vi "Parse XML Tree Example.vi"() -> ()   [LabVIEW 2016]
uses:
  <vilib>/xml/Load XML File.vi
  <vilib>/ni/Tree/Tree Manager/API/List Roots.vi
  <vilib>/ni/Tree/Tree Manager/Tree.lvclass
  <vilib>/xml/NI_XML.lvlib
panel:
  in  "Tree":string(tree)
  out "Error Out":errorcluster
  in  "path to XML document":path
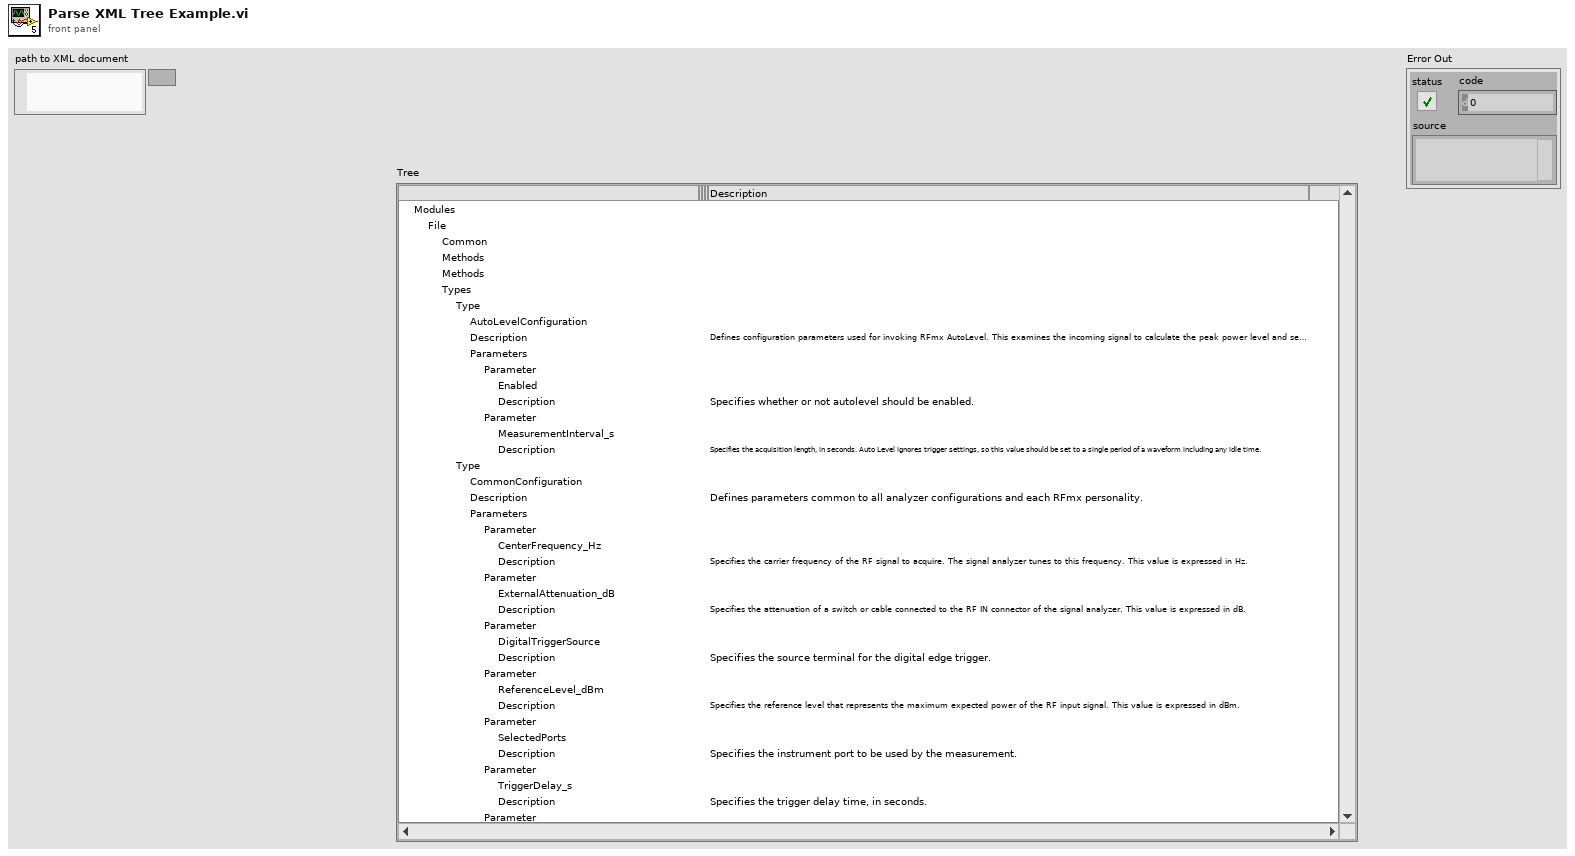
[diagram p1: front panel]
types:
  T1 = cluster{"Left Cell String":string, "Child Text":string[], "Child Tag":string, "Item Indent":i32, "Child Only?":bool, "Glyph Index":i32}[]
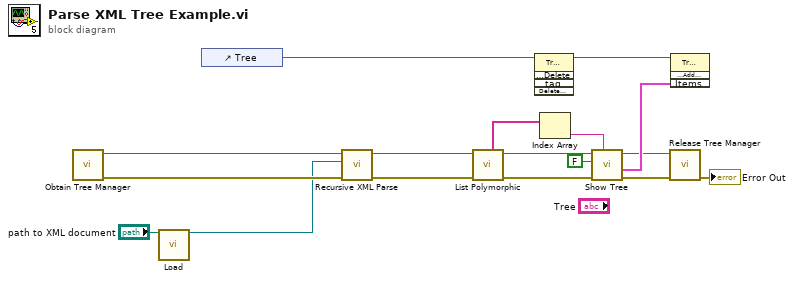
[diagram p0: block diagram]
diagram:
  n1 = call <vilib>:"Obtain Tree Manager.vi"() -> ("Error Out"=w15:errorcluster, "Tree"=w8:refnum<data-value>)  [unwired: 10 in]
  n2 = call-poly <vilib>:"Load.vi"("path to XML document"="path to XML document") -> ("DOM document out"=w1:refnum<k20>)  [unwired: 12 in, 2 out]
  n3 = control-ref of="Tree"() -> (w3:refnum<vi>)
  n4 = call "Recursive XML Parse.vi"("error in (no error)"=w15, "DOM document in"=w1, "Tree"=w8) -> ("error out"=w14:errorcluster, "Tree Manager"=w7:refnum<data-value>)  [unwired: 7 in]
  n5 = call-poly <vilib>:"List Polymorphic.vi"("Error In"=w14, "Tree"=w7) -> ("Error Out"=w13:errorcluster, "Tree"=w12:refnum<data-value>, "Roots IDs"=w4:string[])  [unwired: 6 in, 1 out]
  n6 = invoke class="Tree (strict)" method="Edit Tree Items.Delete"(reference=w3) -> (reference out=w16:refnum<vi>)  [unwired: 4 in, 4 out]
  n7 = Index Array(array=w4) -> (element=w11:string)  [unwired: 1 in]
  n8 = call <vilib>:"Show Tree.vi"("Root ID"=w11, "Error In"=w13, "Show IDs (False)"=FALSE, "Tree"=w12) -> ("Error Out"=w10:errorcluster, "Items Out"=w17:T1, "Tree"=w9:refnum<data-value>)  [unwired: 5 in]
  n9 = call <vilib>:"Release Tree Manager.vi"("Error In"=w10, "Tree"=w9) -> ("Error Out"=→"Error Out":errorcluster)  [unwired: 9 in]
  n10 = invoke class="Tree (strict)" method="Edit Tree Items.Add Multiple Items to End"(reference=w16, "Items"=w17) -> ()  [unwired: 2 in, 4 out]
